vi "PostPersonnel.vi"(8 "error in (no error)":errorcluster, 9 "Data":string, 10 "Commands":T1, 11 "PUID":string) -> (0 "error out":errorcluster, 2 "body":string)   [LabVIEW 2015, in "PersonnelRestApi.lvlib"]
uses:
  PersonnelRestApi.lvlib
  TypeDef/PostPersonnelCommands.ctl
  TypeDef/FGVAction.ctl
  <vilib>/httpClient/POSTBuffer.vi
  <vilib>/httpClient/LabVIEWHTTPClient.lvlib
  RoomRestApi.lvlib
panel:
  out "concatenated string":string
  out "URL":string
  out "headers":string
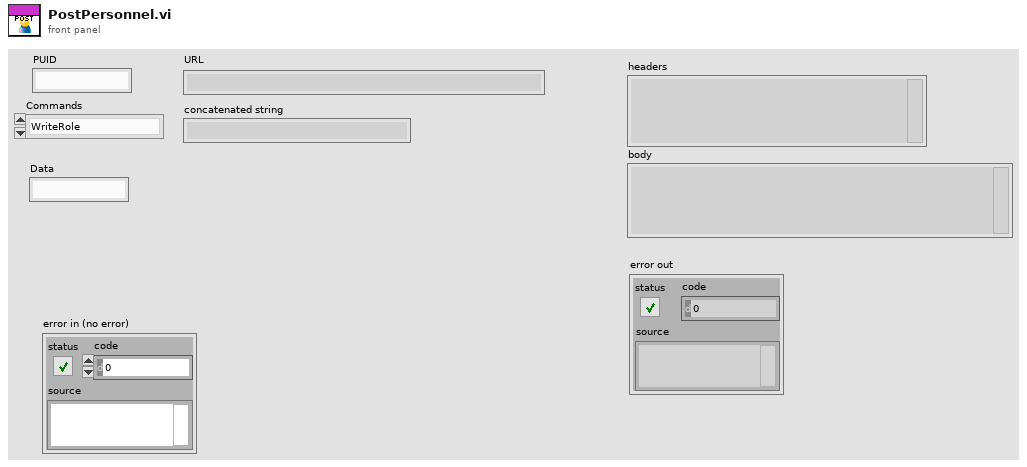
[diagram p1: front panel]
types:
  T1 = typedef "PersonnelRestApi.lvlib/PostPersonnelCommands.ctl" = enum16{"WriteRole", "WriteName", "AddRequest", "RemoveRequest", "IntoRoom", "OutOfRoom", "Register"}
  T2 = typedef "RoomRestApi.lvlib/FGVAction.ctl" = enum16{"Get", "Set"}
  T3 = typedef "LabVIEWHTTPClient.lvlib/ClientHandle.ctl" = refnum<k1>
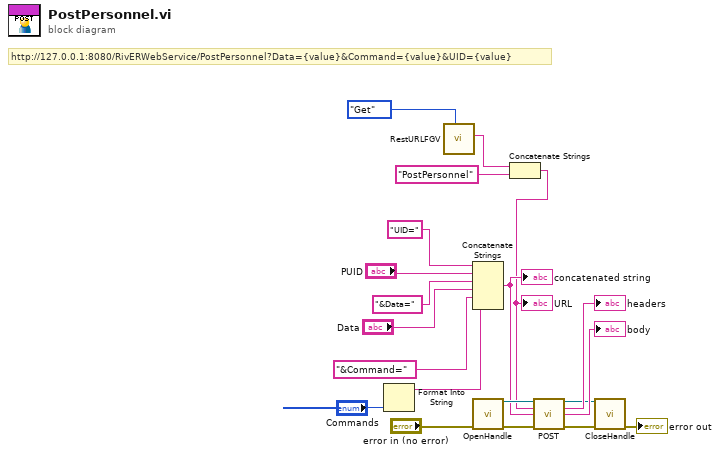
[diagram p0: block diagram]
diagram:
  # "http://127.0.0.1:8080/RivERWebService/PostPersonnel?Data={value}&Command={value}&UID={value}"
  n1 = Format Into String("Commands") -> (resulting string=w4:string)  [unwired: 3 in, 1 out]
  n2 = call "RestURLFGV.vi"("Action"=FGVAction."Get") -> ("URL"=w8:string)  [unwired: 9 in, 1 out]
  n3 = Concatenate Strings("UID=" ("string"), "PUID", "&Data=" ("string"), "Data", "&Command=" ("string"), w4) -> (w11:string)
  "concatenated string" <- w11
  n4 = call <vilib>:"OpenHandle.vi"("error in (no error)"="error in (no error)") -> ("client handle out"=w20:T3, "error out"=w15:errorcluster)  [unwired: 13 in]
  n5 = Concatenate Strings(w8, "PostPersonnel" ("string")) -> (w6:string)
  "URL" <- w6
  n6 = call-poly <vilib>:"POST.vi"("client handle"=w20, "url"=w6, "buffer"=w11, "error in (no error)"=w15) -> ("client handle out"=w17:T3, "headers"=→"headers":string, "body"=→"body":string, "error out"=w16:errorcluster)  [unwired: 8 in]
  n7 = call <vilib>:"CloseHandle.vi"("client handle"=w17, "error in (no error)"=w16) -> ("error out"=→"error out":errorcluster)  [unwired: 13 in]
